vi "Write SolenoidDevRef.vi"(8 "error in (no error)":errorcluster, 10 "SolenoidDevRef":T1={"DevStatus"={"status"=FALSE, "code"=0, "source"=""}, "Solenoid Module"=enum."Solenoid Module 1", "Forward Solenoid Channel"=enum."Invalid", "Reverse Solenoid Channel"=enum."Invalid"}, 11 "Shifter in":refnum<class "Shifter.lvclass">) -> (0 "error out":errorcluster, 3 "Shifter out":refnum<class "Shifter.lvclass">)   [LabVIEW 2013, in "Shifter.lvclass"]
uses:
  Shifter.lvclass
  <vilib>/Rock Robotics/WPI/Solenoid/WPI_SolenoidDevRef.ctl
  <vilib>/Rock Robotics/SystemInterfaces/Typedef/FPGA_TypedefSolenoidModule.ctl
  <vilib>/Rock Robotics/WPI/Solenoid/WPI_SolenoidChannel.ctl
  Shifter.lvclass/Shifter.ctl
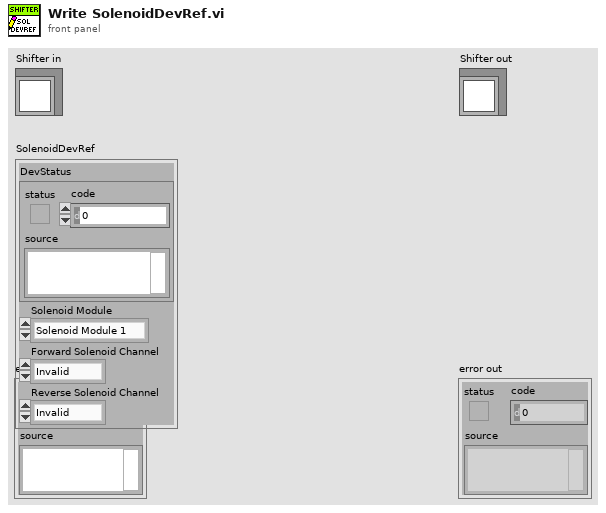
[diagram p1: front panel]
types:
  T1 = typedef "WPI_SolenoidDevRef.ctl" = cluster{"DevStatus":errorcluster, "Solenoid Module":T2, "Forward Solenoid Channel":T3, "Reverse Solenoid Channel":T3}
  T2 = typedef "FPGA_TypedefSolenoidModule.ctl" = enum16{"Solenoid Module 1", "Solenoid Module 2"}
  T3 = typedef "WPI_SolenoidChannel.ctl" = enum8{"Solenoid 1", "Solenoid 2", "Solenoid 3", "Solenoid 4", "Solenoid 5", "Solenoid 6", "Solenoid 7", "Solenoid 8", "Invalid"}
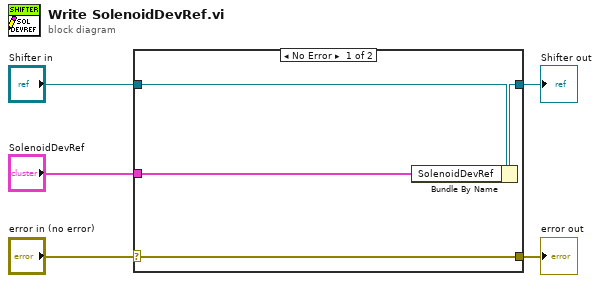
[diagram p0: block diagram]
diagram:
  n1 = case shown="No Error" "error in (no error)" {
    selector: "error in (no error)" -> [w9 w10]
    tunnel: [w9 w10] -> w4
    tunnel: [w7 w11] -> w2
    tunnel: "Shifter in" -> [w8 w11]
    tunnel: "SolenoidDevRef" -> [w6 _]
    frame No Error {
      n2 = Bundle By Name(cluster=w8, "SolenoidDevRef"=w6) -> (w7:refnum<class "Shifter.lvclass">)
    }
    frame Error {
    }
  }
  "error out" <- w4
  "Shifter out" <- w2
